vi "removeSheet.vi"(8 "error in (no error)":errorcluster, 10 "Sheet Index":i32, 11 "MS-Excel in":refnum<class "MS-Excel.lvclass">) -> (0 "error out":errorcluster, 3 "MS-Excel out":refnum<class "MS-Excel.lvclass">)   [LabVIEW 2017, in "LabVIEW NPOI.lvlib" / "MS-Excel.lvclass"]
uses:
  MS-Excel.lvclass
  D:/Benjamin/Documents/Perso/Code/WC/LabVIEW_NPOI/lib/NPOI 2.1.1/NPOI.dll
  lib/NPOI 2.1.1/NPOI.dll
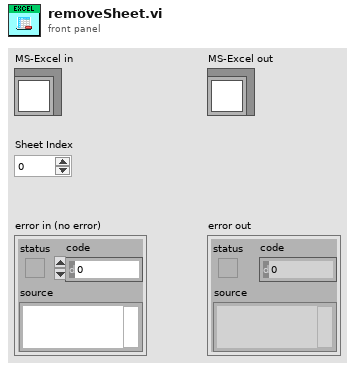
[diagram p1: front panel]
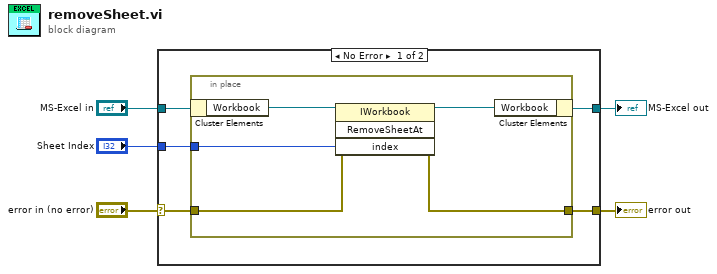
[diagram p0: block diagram]
diagram:
  n1 = case shown="No Error" "error in (no error)" {
    selector: "error in (no error)" -> [w7 w16]
    tunnel: [w6 w16] -> w5
    tunnel: [w10 w17] -> w3
    tunnel: "MS-Excel in" -> [w9 w17]
    tunnel: "Sheet Index" -> [w8 _]
    frame No Error {
      n2 = in-place {
        in-place-border: w8 -> [w13]
        in-place-border: w7 -> [w12]
        in-place-border: [w11] -> w6
        n3 = in-place-cluster #1(w9) -> ("Workbook"=w15:refnum<k24>)
        n4 = invoke class="IWorkbook" method="RemoveSheetAt"(reference=w15, error in=w12, "index"=w13) -> (reference out=w14:refnum<k24>, error out=w11:errorcluster)  [unwired: 1 in, 2 out]
        n5 = in-place-cluster #1("Workbook"=w14) -> (w10:refnum<class "MS-Excel.lvclass">)
      }
    }
    frame Error {
    }
  }
  "error out" <- w5
  "MS-Excel out" <- w3
